vi "Rx Ch Start.vi"(10 "Channel":u8, 11 "devId":i32) -> (2 "devId out":i32, 3 "function return":i32)   [LabVIEW 2013, in "CHR34XXX.lvlib"]
doc: "DLL BOOL __stdcall CHR34XXX_RxCh_ClearOFFlag(IN int devId,IN BYTE Channel); DLL BOOL __stdcall CHR34XXX_RxCh_ClearFIFO(IN int devId,IN BYTE Channel); DLL BOOL __stdcall CHR34XXX_RxCh_Start(IN int devId,IN BYTE Channel);"
uses:
  CHR34XXX.lvlib
  CHR34XXX.dll
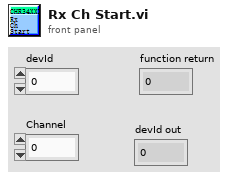
[diagram p1: front panel]
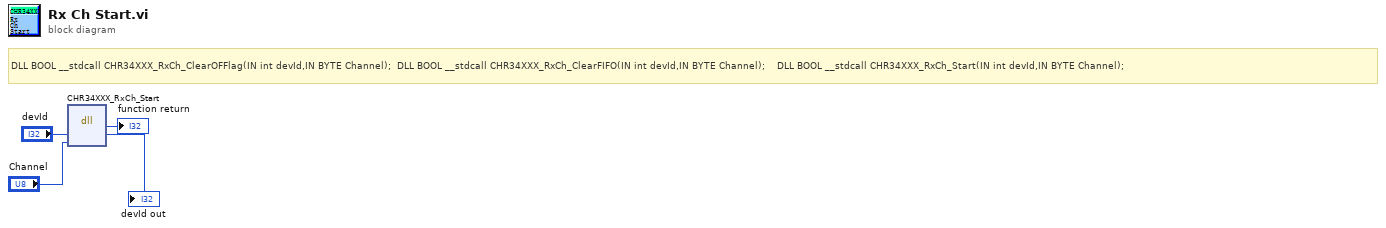
[diagram p0: block diagram]
diagram:
  # "DLL BOOL __stdcall CHR34XXX_RxCh_ClearOFFlag(IN int devId,IN BYTE Channel);  DLL BOOL __stdcall CHR34XXX_RxCh_ClearFIFO(IN int devId,IN BYTE Channel);    DLL BOOL __stdcall CHR34XXX_RxCh_Start(IN int devId,IN BYTE Channel);"
  n1 = dll-call lib="C:/Users/dy/Desktop/CHR34XXX_lv/lv_lib/CHR34XXX.*" fn="CHR34XXX_RxCh_Start"("devId"="devId", "Channel"="Channel") -> (→"function return":i32, "devId"=→"devId out":i32)  [unwired: 4 in, 2 out]
